vi "Output_DL.vi"(7 "Private Data":refnum<class "DataLogger.lvclass">, 8 "error in (no error)":errorcluster, 10 "OutputCluster":T1, 11 "State":string) -> (0 "error out":errorcluster)   [LabVIEW 2019, in "DataLogger.lvclass"]
doc: "Output_DL"
uses:
  DataLogger.lvclass
  <vilib>/ActorFramework/Actor/Actor.lvclass
  Inspection Statemachine/Inspection Statemachine Messages/Acknowledgement_SM Msg/Acknowledgement_SM.lvclass
  Inspection Statemachine/Inspection Statemachine Messages/ButtonPressed_SM Msg/ButtonPressed_SM Msg.lvclass
  Inspection Statemachine/Inspection Statemachine Messages/ErrorMessage_SM Msg/ErrorMessage_SM Msg.lvclass
  C:/Program Files/National Instruments/LabVIEW 2019/vi.lib/ActorFramework/Actor/Actor.lvclass
  <vilib>/ActorFramework/Message Enqueuer/Message Enqueuer.lvclass
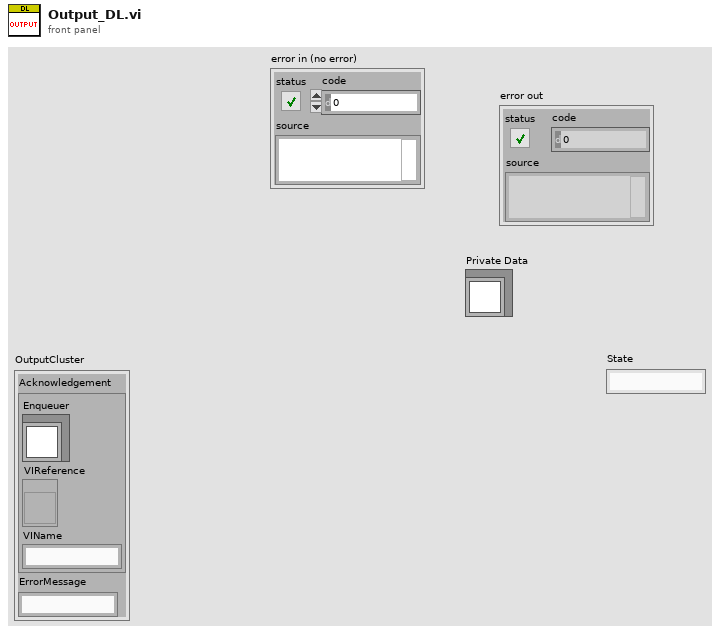
[diagram p1: front panel]
types:
  T1 = cluster{"Acknowledgement":cluster{"Enqueuer":refnum<class "Message Enqueuer.lvclass">, "VIReference":refnum<vi>, "VIName":string}, "ErrorMessage":string}
  T2 = cluster{"Enqueuer":refnum<class "Message Enqueuer.lvclass">, "VIReference":refnum<vi>, "VIName":string}
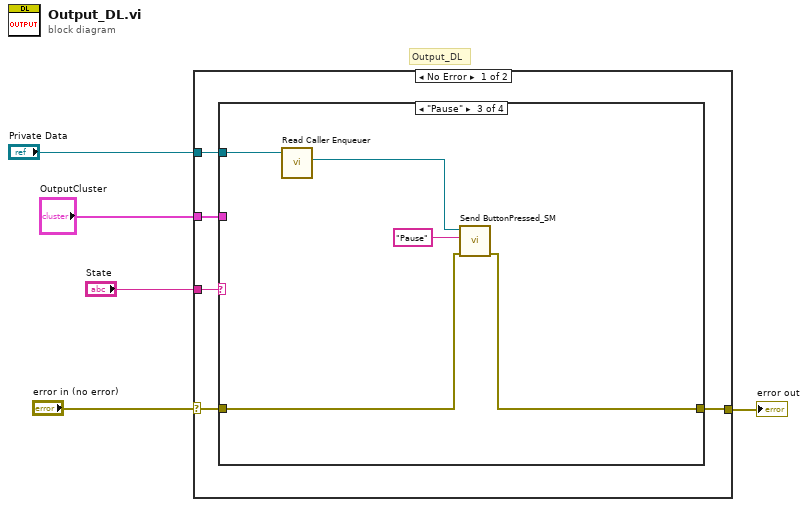
[diagram p0: block diagram]
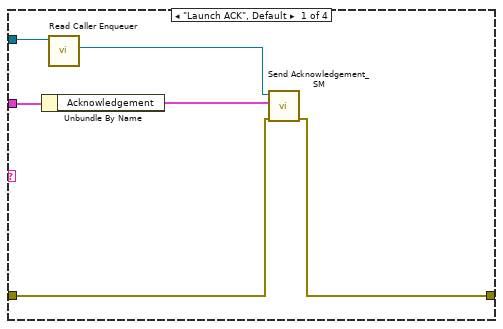
[diagram p2: hidden frame]
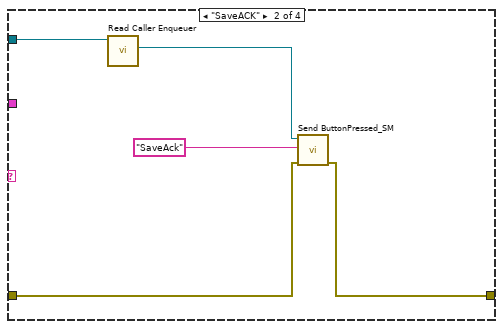
[diagram p3: hidden frame]
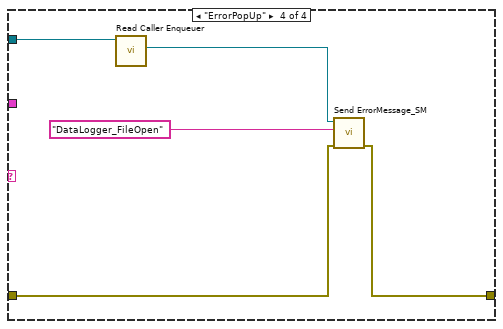
[diagram p4: hidden frame]
diagram:
  # "Output_DL"
  n1 = case shown="No Error" "error in (no error)" {
    selector: "error in (no error)" -> [w7 w32]
    tunnel: "State" -> [w10 _]
    tunnel: "Private Data" -> [w9 _]
    tunnel: "OutputCluster" -> [w8 _]
    tunnel: [w6 w32] -> w2
    frame No Error {
      n2 = case shown="\"Pause\"" w10 {
        tunnel: w9 -> [w16 w21 w26 w31]
        tunnel: w8 -> [w12 _ _ _]
        tunnel: w7 -> [w15 w20 w23 w30]
        tunnel: [w14 w19 w22 w29] -> w6
        frame "Launch ACK", Default {
          n3 = Unbundle By Name(w12) -> ("Acknowledgement"=w11:T2)
          n4 = call <vilib>:"Read Caller Enqueuer.vi"("Actor"=w16) -> ("Caller Enqueuer"=w13:refnum<class "Message Enqueuer.lvclass">)  [unwired: 10 in]
          n5 = call "Send Acknowledgement_SM.vi"("error in (no error)"=w15, "Acknowledgement"=w11, "Message Enqueuer"=w13) -> ("error out"=w14:errorcluster)  [unwired: 7 in, 1 out]
        }
        frame "SaveACK" {
          n6 = call <vilib>:"Read Caller Enqueuer.vi"("Actor"=w21) -> ("Caller Enqueuer"=w17:refnum<class "Message Enqueuer.lvclass">)  [unwired: 10 in]
          n7 = call "Send ButtonPressed_SM.vi"("error in (no error)"=w20, "ButtonPress"="SaveAck", "Message Enqueuer"=w17) -> ("error out"=w19:errorcluster)  [unwired: 7 in, 1 out]
        }
        frame "Pause" {
          n8 = call <vilib>:"Read Caller Enqueuer.vi"("Actor"=w26) -> ("Caller Enqueuer"=w25:refnum<class "Message Enqueuer.lvclass">)  [unwired: 10 in]
          n9 = call "Send ButtonPressed_SM.vi"("error in (no error)"=w23, "ButtonPress"="Pause", "Message Enqueuer"=w25) -> ("error out"=w22:errorcluster)  [unwired: 7 in, 1 out]
        }
        frame "ErrorPopUp" {
          n10 = call <vilib>:"Read Caller Enqueuer.vi"("Actor"=w31) -> ("Caller Enqueuer"=w28:refnum<class "Message Enqueuer.lvclass">)  [unwired: 10 in]
          n11 = call "Send ErrorMessage_SM.vi"("error in (no error)"=w30, "Error Message"="DataLogger_FileOpen", "Message Enqueuer"=w28) -> ("error out"=w29:errorcluster)  [unwired: 7 in, 1 out]
        }
      }
    }
    frame Error {
    }
  }
  "error out" <- w2
